vi "Run Core.vi"(8 "Error In":errorcluster, 9 "Timeout (s)":dbl, 10 "ConfigA In":refnum<class "ConfigA.lvclass">, 11 "Reference In":refnum<class "IDMM.lvclass">) -> (0 "Error Out":errorcluster, 1 "Timeout?":bool, 2 "IResult Out":refnum<class "IResult.lvclass">, 3 "Reference Out":refnum<class "IDMM.lvclass">)   [LabVIEW 2020, in "ConfigA.lvclass"]
uses:
  ConfigA.lvclass
  IReference/IDMM.lvclass
  IResult/IResult.lvclass
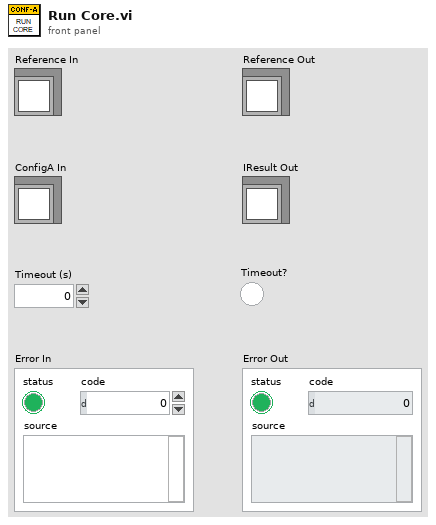
[diagram p1: front panel]
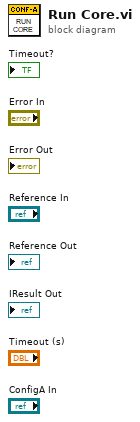
[diagram p0: block diagram]
diagram:
